vi "GetLastSelectedRowIndex.vi"(0 "reference in":refnum<class "DataGridView.lvclass">, 11 "error in (no error)":errorcluster) -> (4 "reference out":refnum<class "DataGridView.lvclass">, 6 "LastSelectedRowIndex":i32=-1, 15 "error out":errorcluster)   [LabVIEW 2018, in "DataGridView.lvclass"]
doc: "Gets the last selected index, if nothing was selected it returns -1"
uses:
  DataGridView.lvclass
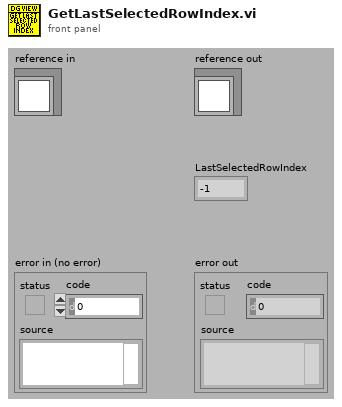
[diagram p1: front panel]
types:
  T1 = typedef "DataGridView.lvclass/ObjectAttributes.ctl" = cluster{"DataGridView":refnum<k24>, "SelectionChangedEvent":refnum<user-event>, "SelectionChanged callback ref":refnum<k27>, "LastSelectedRowIndex":i32}
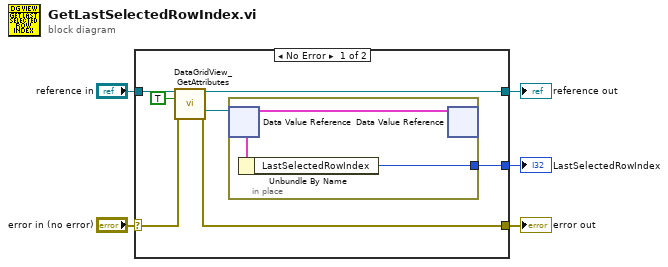
[diagram p0: block diagram]
diagram:
  n1 = case shown="No Error" "error in (no error)" {
    selector: "error in (no error)" -> [w12 w16]
    tunnel: [w11 w16] -> w4
    tunnel: [w9 w15] -> w2
    tunnel: "reference in" -> [w10 w15]
    tunnel: [w8 _] -> w1
    frame No Error {
      n2 = call "DataGridView_GetAttributes.vi"("reference in"=w10, "OnlyGetDvrReference(False)"=TRUE, "error in (no error)"=w12) -> ("reference out"=w9:refnum<class "DataGridView.lvclass">, "DataRef"=w6:refnum<data-value>, "error out"=w11:errorcluster)  [unwired: 9 in, 1 out]
      n3 = in-place {
        in-place-border: [w14] -> w8
        n4 = in-place-dvr #1(w6) -> (w13:T1)  [unwired: 1 out]
        n5 = Unbundle By Name(w13) -> ("LastSelectedRowIndex"=w14:i32)
        n6 = in-place-dvr #1(w13) -> ()  [unwired: 2 out]
      }
    }
    frame Error {
    }
  }
  "error out" <- w4
  "reference out" <- w2
  "LastSelectedRowIndex" <- w1
